vi "PH_Beckhoff.set Digital Outputs Defaults.vi"(1 "Service IDs":i32[](array[numeric]), 2 "inverted?":bool[](array[boolean]), 3 "Digital Output Tag Names":string[](array[string])) -> (0 "Digital Outputs":T2)   [LabVIEW 2014, in "PH_Beckhoff.lvlib"]
uses:
  PH_Beckhoff.lvlib
  PH_Beckhoff.Digital Outputs.ctl
panel:
  in  "Digital Output Value":T1
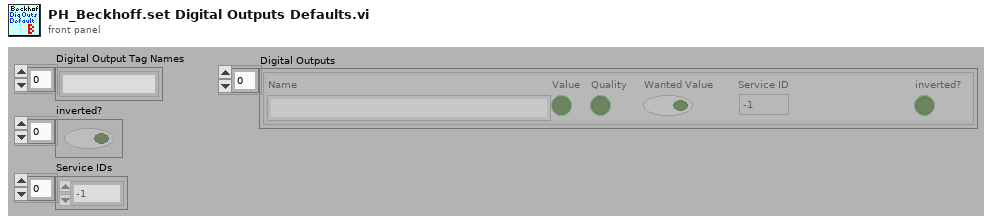
[diagram p1: front panel]
types:
  T1 = cluster{"Name":string, "Value":bool, "Quality":bool, "Wanted Value":bool, "Service ID":i32, "inverted?":bool}
  T2 = typedef "PH_Beckhoff.lvlib/PH_Beckhoff.Digital Outputs.ctl" = cluster{"Name":string, "Value":bool, "Quality":bool, "Wanted Value":bool, "Service ID":i32, "inverted?":bool}[]
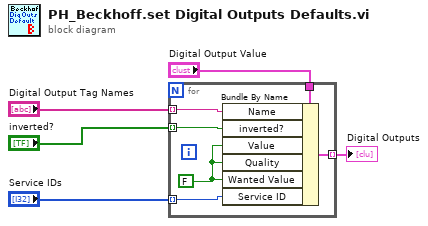
[diagram p0: block diagram]
diagram:
  n1 = for {
    tunnel: "Digital Output Value" -> [w11]
    tunnel: [w10] -> w4 mode=indexing
    tunnel: "Digital Output Tag Names" -> [w9] mode=indexing
    tunnel: "inverted?" -> [w8] mode=indexing
    tunnel: "Service IDs" -> [w6] mode=indexing
    w7 = FALSE ("Quality")
    n2 = Bundle By Name(cluster=w11, "Name"=w9, "inverted?"=w8, "Value"=w7, "Quality"=w7, "Wanted Value"=w7, "Service ID"=w6) -> (w10:T1)
  }
  "Digital Outputs" <- w4
